vi "Read Display - Format String.vi"(8 "error in (no error)":errorcluster, 11 "NT Scalar (Numeric) in":refnum<class "NT Scalar (Numeric).lvclass">) -> (0 "error out":errorcluster, 2 "format string":string, 3 "NT Scalar (Numeric) out":refnum<class "NT Scalar (Numeric).lvclass">)   [LabVIEW 2020, in "PV Access.lvlib" / "PV Data.lvlib" / "NT Scalar (Numeric).lvclass"]
uses:
  NT Scalar (Numeric).lvclass
  NT Scalar (Numeric).lvclass/NT Scalar (Numeric).ctl
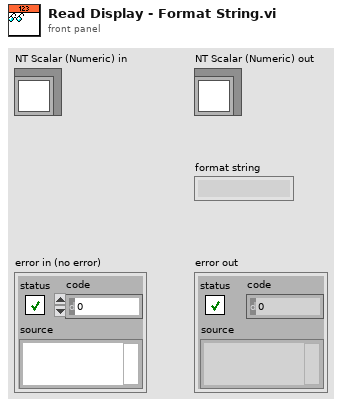
[diagram p1: front panel]
types:
  T1 = typedef "PV Access.lvlib/PV Data.lvlib/Display Form.ctl" = enum16{"Default", "String", "Binary", "Decimal", "Hex", "Exponential", "Engineering"}
  T2 = typedef "PV Access.lvlib/PV Data.lvlib/Type Code.ctl" = enum8{"Null", "Bool", "BoolA", "Int8", "Int8A", "Int16", "Int16A", "Int32", "Int32A", "Int64", "Int64A", "UInt8", "UInt8A", "UInt16", "UInt16A", "UInt32", "UInt32A", "UInt64", "UInt64A", "Float32", "Float32A", "Float64", "Float64A", "String", "StringA", "Struct", "StructA", "Union", "UnionA", "Any", "AnyA"}
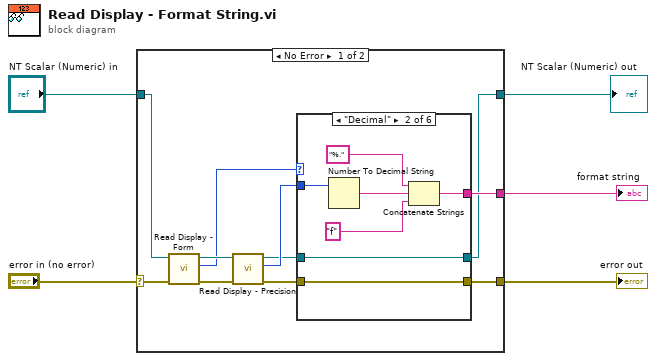
[diagram p0: block diagram]
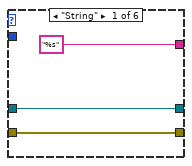
[diagram p2: hidden frame]
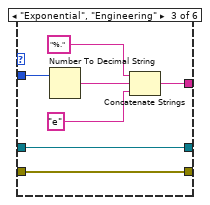
[diagram p3: hidden frame]
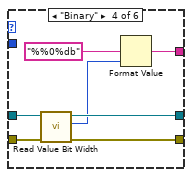
[diagram p4: hidden frame]
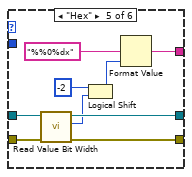
[diagram p5: hidden frame]
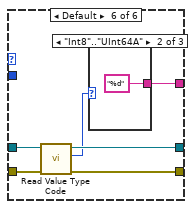
[diagram p6: hidden frame]
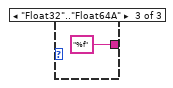
[diagram p8: hidden frame]
diagram:
  n1 = case shown="No Error" "error in (no error)" {
    selector: "error in (no error)" -> [w15 w58]
    tunnel: [w8 w58] -> w4
    tunnel: [w6 w59] -> w2
    tunnel: "NT Scalar (Numeric) in" -> [w13 w59]
    tunnel: [w16 _] -> w1
    frame No Error {
      n2 = call-dynamic "Read Display - Form.vi"("error in (no error)"=w15, "NT Scalar (Numeric) in"=w13) -> ("error out"=w14:errorcluster, "form"=w11:T1, "NT Scalar (Numeric) out"=w12:refnum<class "NT Scalar (Numeric).lvclass">)  [unwired: 7 in]
      n3 = call-dynamic "Read Display - Precision.vi"("error in (no error)"=w14, "NT Scalar (Numeric) in"=w12) -> ("error out"=w9:errorcluster, "precision"=w10:i32, "NT Scalar (Numeric) out"=w7:refnum<class "NT Scalar (Numeric).lvclass">)  [unwired: 7 in]
      n4 = case shown="\"Decimal\"" w11 {
        tunnel: w10 -> [_ w26 w33 _ _ _]
        tunnel: ["%s" w25 w31 w35 w48 w50] -> w16
        tunnel: w9 -> [w17 w21 w27 w40 w47 w55]
        tunnel: [w17 w21 w27 w38 w46 w54] -> w8
        tunnel: w7 -> [w18 w20 w28 w39 w45 w53]
        tunnel: [w18 w20 w28 w37 w44 w52] -> w6
        frame "String" {
        }
        frame "Decimal" {
          n5 = Number To Decimal String(number=w26) -> (decimal integer string=w24:string)  [unwired: 1 in]
          n6 = Concatenate Strings("%.", w24, "f") -> (w25:string)
        }
        frame "Exponential", "Engineering" {
          n7 = Number To Decimal String(number=w33) -> (decimal integer string=w30:string)  [unwired: 1 in]
          n8 = Concatenate Strings("%.", w30, "e") -> (w31:string)
        }
        frame "Binary" {
          n9 = call "Read Value Bit Width.vi"("error in (no error)"=w40, "NT Scalar (Numeric) in"=w39) -> ("error out"=w38:errorcluster, "value bit width"=w34:i32, "NT Scalar (Numeric) out"=w37:refnum<class "NT Scalar (Numeric).lvclass">)  [unwired: 7 in]
          n10 = Format Value(format string="%%0%db", value (0)=w34) -> (output string=w35:string)  [unwired: 1 in]
        }
        frame "Hex" {
          n11 = call "Read Value Bit Width.vi"("error in (no error)"=w47, "NT Scalar (Numeric) in"=w45) -> ("error out"=w46:errorcluster, "value bit width"=w41:i32, "NT Scalar (Numeric) out"=w44:refnum<class "NT Scalar (Numeric).lvclass">)  [unwired: 7 in]
          n12 = Logical Shift(y=-2 ("x"), x=w41) -> (x << y=w42:i32)
          n13 = Format Value(format string="%%0%dx", value (0)=w42) -> (output string=w48:string)  [unwired: 1 in]
        }
        frame Default {
          n14 = call-dynamic "Read Value Type Code.vi"("error in (no error)"=w55, "NT Scalar in"=w53) -> ("error out"=w54:errorcluster, "type code"=w51:T2, "NT Scalar out"=w52:refnum<class "NT Scalar (Numeric).lvclass">)  [unwired: 7 in]
          n15 = case shown="\"Int8\"..\"UInt64A\"" w51 {
            tunnel: [_ "%d" "%f"] -> w50
            frame Default {
            }
            frame "Int8".."UInt64A" {
            }
            frame "Float32".."Float64A" {
            }
          }
        }
      }
    }
    frame Error {
    }
  }
  "error out" <- w4
  "NT Scalar (Numeric) out" <- w2
  "format string" <- w1
